vi "WorkorderHandler_LatestSr.vi"(8 "error in (no error)":errorcluster, 11 "reference":T1) -> (0 "error out":errorcluster, 1 "Bad":string, 2 "OK":string, 3 "duplicate reference":T1, 5 "SrNo":string)   [LabVIEW 2011]
uses:
  DataStructures/WorkorderHandler_ObjectReference.ctl
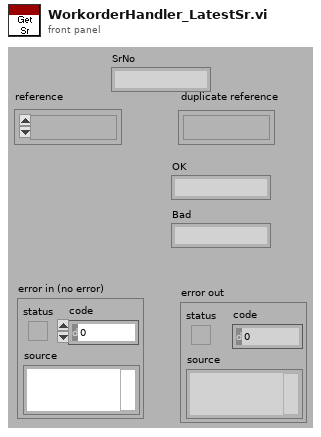
[diagram p1: front panel]
types:
  T1 = typedef "WorkorderHandler_ObjectReference.ctl" = refnum<k1>
  T2 = typedef "WorkorderHandler_ObjectData.ctl" = cluster{"Table":string[][], "Script":string, "Order":string, "No":string, "Time":dbl}
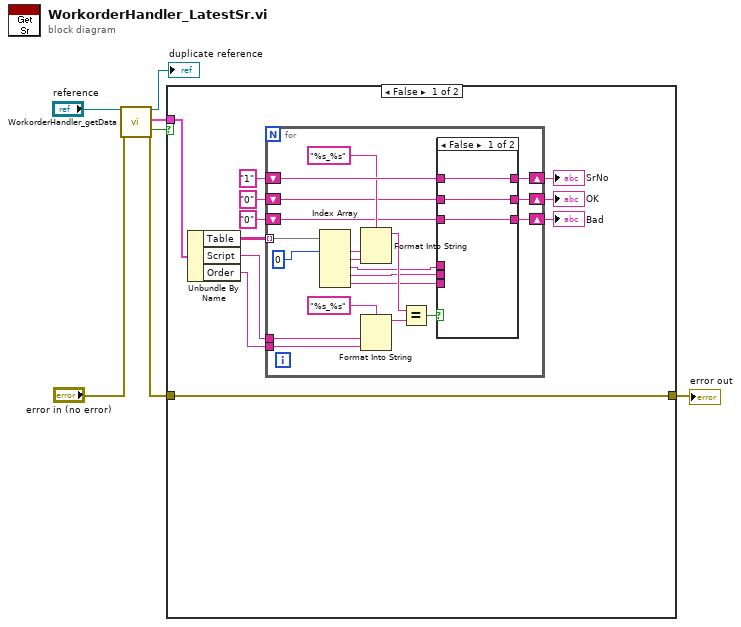
[diagram p0: block diagram]
diagram:
  n1 = call "WorkorderHandler_getData.vi"("reference"="reference", "error in (no error)"="error in (no error)") -> ("duplicate reference"=→"duplicate reference":T1, "data"=w5:T2, "timed out?"=w1:bool, "error out"=w2:errorcluster)  [unwired: 1 in, 13 out]
  n2 = case shown="False" w1 {
    tunnel: w5 -> [w18 _]
    tunnel: [w17 w45] -> w4
    tunnel: w2 -> [w17 w45]
    frame False {
      n3 = Unbundle By Name(w18) -> ("Table"=w16:string[][], "Script"=w15:string, "Order"=w14:string)
      n4 = for {
        tunnel: w16 -> [w38] mode=indexing
        tunnel: w15 -> [w29]
        shift-right: [w34] -> w12
        shift-left: "1" ("String") -> [w35]
        tunnel: w14 -> [w28]
        shift-right: [w24] -> w11
        shift-left: "0" ("String") -> [w23]
        shift-right: [w21] -> w8
        shift-left: "0" ("String") -> [w22]
        n5 = Index Array(array=w38, index #1=0 ("index")) -> (element #1=w31:string, element #2=w30:string, element #3=w25:string, element #4=w20:string, element #5=w19:string)  [unwired: 4 in]
        n6 = Format Into String(format string="%s_%s", w31, w30) -> (resulting string=w27:string)  [unwired: 2 in, 1 out]
        n7 = Format Into String(format string="%s_%s", w29, w28) -> (resulting string=w26:string)  [unwired: 2 in, 1 out]
        n8 = Equal?(x=w27, y=w26) -> (x = y?=w36:bool)
        n9 = case shown="False" w36 {
          tunnel: w35 -> [w41 _]
          tunnel: [w41 w44] -> w34
          tunnel: w25 -> [_ w44]
          tunnel: w23 -> [w40 _]
          tunnel: [w40 w43] -> w24
          tunnel: w22 -> [w39 _]
          tunnel: [w39 w42] -> w21
          tunnel: w20 -> [_ w43]
          tunnel: w19 -> [_ w42]
          frame False {
          }
          frame True {
          }
        }
      }
      "SrNo" <- w12
      "OK" <- w11
      "Bad" <- w8
    }
    frame True {
      # "Error or Timed Out"
    }
  }
  "error out" <- w4
